vi "Notifier Test.vi"() -> ()   [LabVIEW 2021]
panel:
  in  "Any":bool
  out "size(s)":i32
  in  "name":string
  out "error out 3":errorcluster
  out "error out 2":errorcluster
  out "error out":errorcluster
  out "Iterations":i32
  in  "Add":bool
  in  "stop 2":bool
  in  "Send one":bool
  in  "Send two":bool
  in  "stop":bool
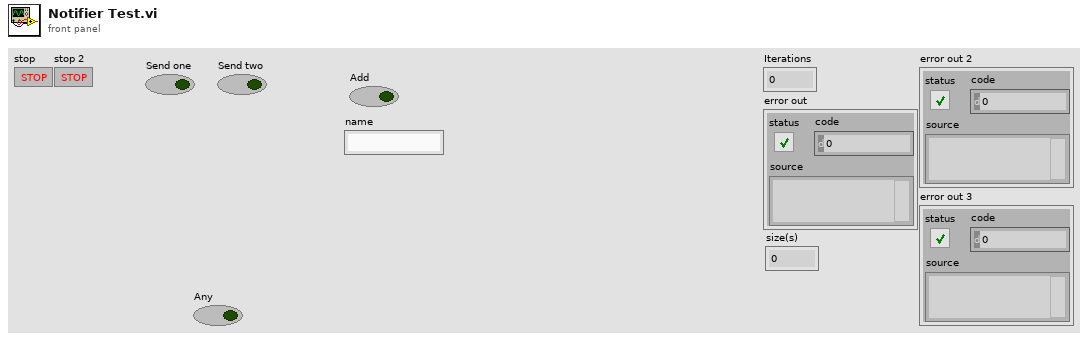
[diagram p1: front panel]
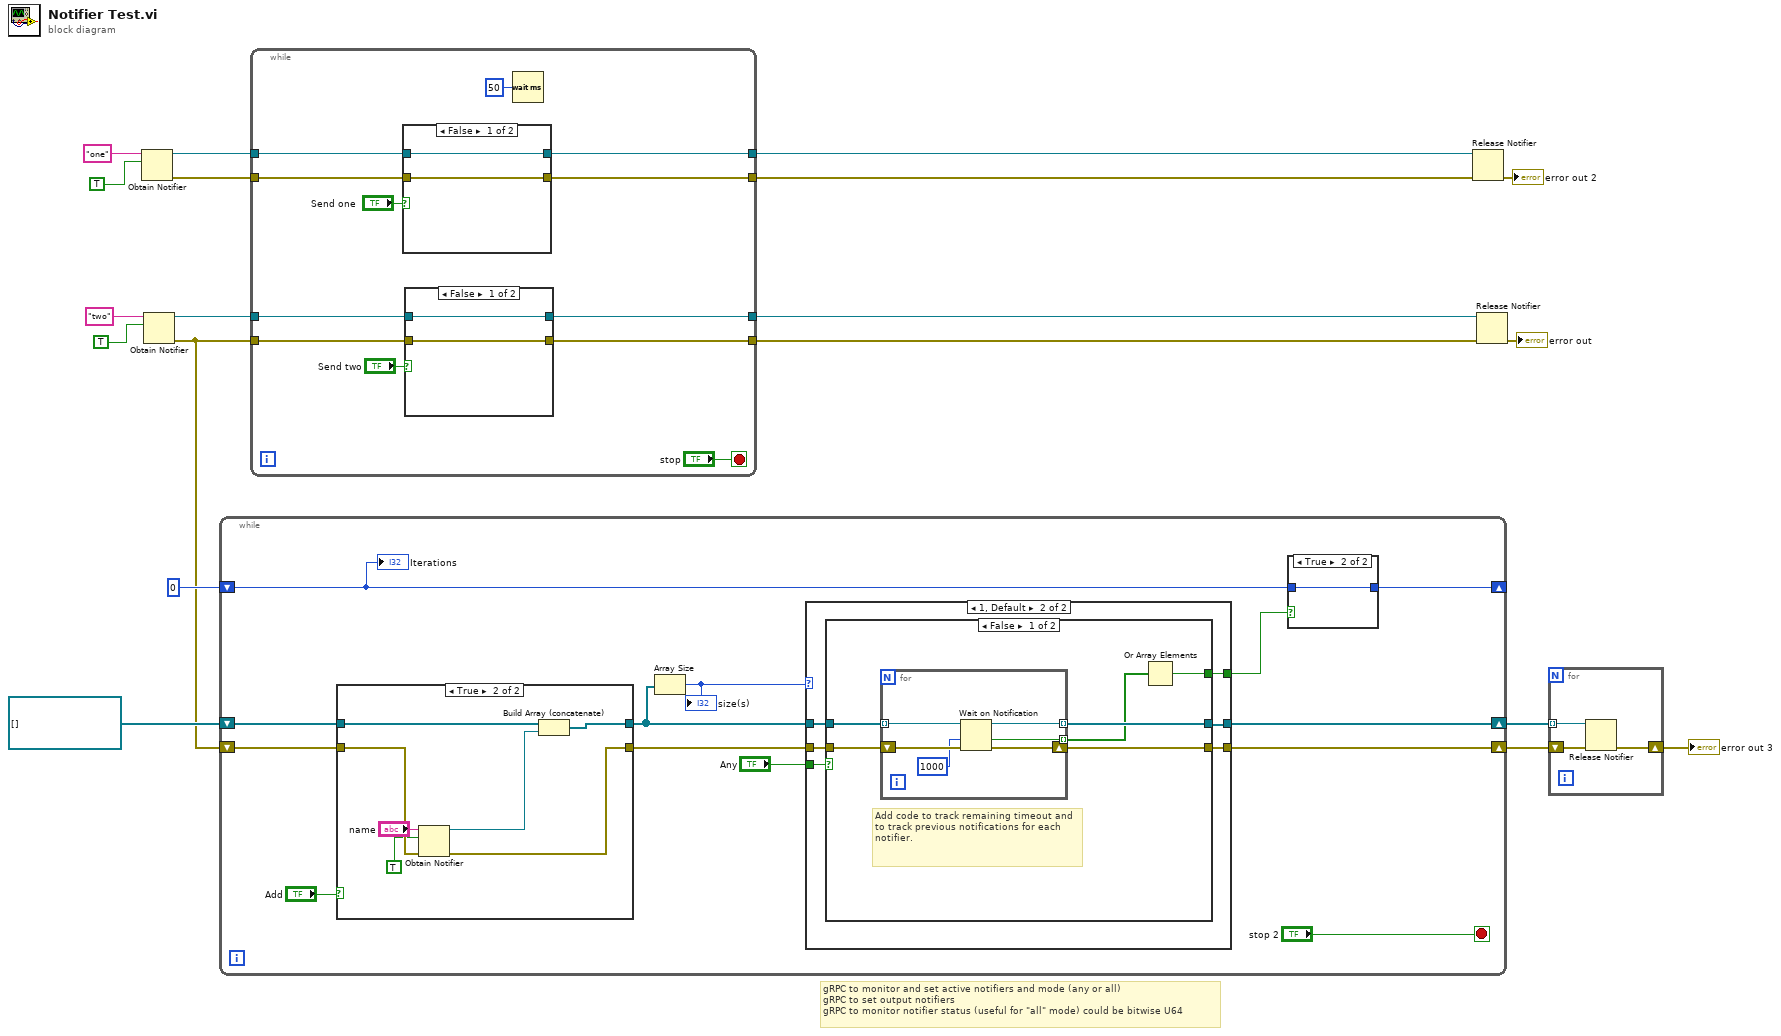
[diagram p0: block diagram]
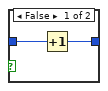
[diagram p2: hidden frame]
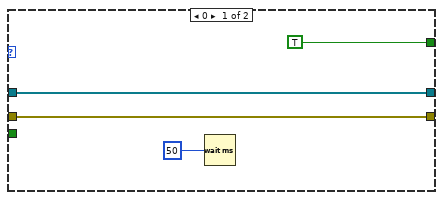
[diagram p3: hidden frame]
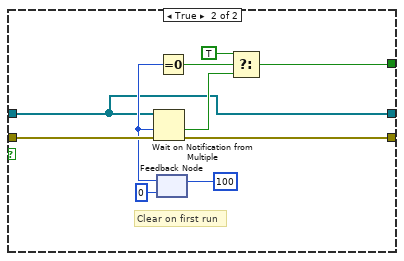
[diagram p4: hidden frame]
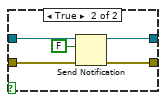
[diagram p6: hidden frame]
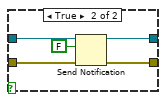
[diagram p7: hidden frame]
diagram:
  # "gRPC to monitor and set active notifiers and mode (any or all)\ngRPC to set output notifiers\ngRPC to monitor notifier status (useful for \"all\" mode) could be bitwise U64"
  n1 = Obtain Notifier(name (unnamed)="one", notification data type=TRUE) -> (notifier out=w14:refnum<notifier>, error out=w13:errorcluster)  [unwired: 2 in, 1 out]
  n2 = Obtain Notifier(name (unnamed)="two", notification data type=TRUE) -> (notifier out=w15:refnum<notifier>, error out=w3:errorcluster)  [unwired: 2 in, 1 out]
  n3 = while {
    shift-right: [w29] -> w6
    shift-left: refnum<notifier>[] [] ("notifiers") -> [w24]
    shift-right: [w21] -> _
    shift-left: 0 -> [w28]
    shift-right: [w27] -> w2
    shift-left: w3 -> [w25]
    stop <- "stop 2" stop-if-true
    n4 = case shown="True" "Add" {
      tunnel: w24 -> [w68 w74]
      tunnel: [w68 w73] -> w23
      tunnel: [w69 w71] -> w26
      tunnel: w25 -> [w69 w76]
      frame False {
      }
      frame True {
        n5 = Obtain Notifier(name (unnamed)="name", notification data type=TRUE, error in (no error)=w76) -> (notifier out=w70:refnum<notifier>, error out=w71:errorcluster)  [unwired: 1 in, 1 out]
        n6 = Build Array (concatenate)(w74, w70) -> (w73:refnum<notifier>[])
      }
    }
    n7 = Array Size(array=w23) -> (size(s)=w30:i32)
    "size(s)" <- w30
    n8 = case shown="1, Default" w30 {
      tunnel: w23 -> [w37 w43]
      tunnel: [w37 w40] -> w29
      tunnel: [w38 w45] -> w27
      tunnel: w26 -> [w38 w44]
      tunnel: [TRUE ("timed out?") w42] -> w22
      tunnel: "Any" -> [_ w41]
      frame 0 {
        n9 = Wait (ms)(milliseconds to wait=u32 50) -> ()  [unwired: 1 out]
      }
      frame 1, Default {
        n10 = case shown="False" w41 {
          tunnel: [w48 w67] -> w45
          tunnel: w44 -> [w50 w66]
          tunnel: w43 -> [w51 w58]
          tunnel: [w47 w59] -> w42
          tunnel: [w49 w58] -> w40
          frame False {
            # "Add code to track remaining timeout and to track previous notifications for each notifier."
            n11 = for {
              tunnel: w51 -> [w56] mode=indexing
              tunnel: [w57] -> w46 mode=indexing
              tunnel: [w55] -> w49 mode=indexing
              shift-right: [w53] -> w48
              shift-left: w50 -> [w54]
              n12 = Wait on Notification(notifier=w56, timeout in ms (-1)=1000, error in (no error)=w54) -> (notifier out=w55:refnum<notifier>, timed out?=w57:bool, error out=w53:errorcluster)  [unwired: 1 in, 1 out]
            }
            n13 = Or Array Elements(Boolean array=w46) -> (logical OR=w47:bool)
          }
          frame True {
            # "Clear on first run"
            n14 = feedback #1(0 ("timeout in ms (-1)")) -> (w63:i32)
            n15 = Wait on Notification from Multiple(0:w58, 2:w63, 3:w66) -> (10:w61:bool, 11:w67:errorcluster)  [unwired: 1 in, 2 out]
            n16 = feedback-in #1(100 ("timeout in ms (-1)")) -> ()
            n17 = Equal To 0?(x=w63) -> (x = 0?=w62:bool)
            n18 = Select(t=TRUE, s=w62, f=w61) -> (s? t:f=w59:bool)
          }
        }
      }
    }
    n19 = case shown="True" w22 {
      tunnel: w28 -> [w34 w35]
      tunnel: [w33 w35] -> w21
      frame False {
        n20 = Increment(x=w34) -> (x+1=w33:i32)
      }
      frame True {
      }
    }
    "Iterations" <- w28
  }
  n21 = while {
    tunnel: [w88] -> w12
    tunnel: [w87] -> w11
    tunnel: w15 -> [w84]
    tunnel: w3 -> [w83]
    tunnel: w14 -> [w80]
    tunnel: w13 -> [w81]
    tunnel: [w79] -> w10
    tunnel: [w78] -> w9
    stop <- "stop" stop-if-true
    n22 = case shown="False" "Send one" {
      tunnel: w80 -> [w90 w95]
      tunnel: w81 -> [w89 w94]
      tunnel: [w90 w93] -> w79
      tunnel: [w89 w92] -> w78
      frame False {
      }
      frame True {
        n23 = Send Notification(notification=FALSE, notifier=w95, error in (no error)=w94) -> (notifier out=w93:refnum<notifier>, error out=w92:errorcluster)
      }
    }
    n24 = case shown="False" "Send two" {
      tunnel: w84 -> [w97 w102]
      tunnel: w83 -> [w96 w101]
      tunnel: [w97 w100] -> w88
      tunnel: [w96 w99] -> w87
      frame False {
      }
      frame True {
        n25 = Send Notification(notification=FALSE, notifier=w102, error in (no error)=w101) -> (notifier out=w100:refnum<notifier>, error out=w99:errorcluster)
      }
    }
    n26 = Wait (ms)(milliseconds to wait=u32 50) -> ()  [unwired: 1 out]
  }
  n27 = Release Notifier(notifier=w10, error in (no error)=w9) -> (error out=→"error out 2":errorcluster)  [unwired: 1 in, 2 out]
  n28 = Release Notifier(notifier=w12, error in (no error)=w11) -> (error out=→"error out":errorcluster)  [unwired: 1 in, 2 out]
  n29 = for {
    tunnel: w6 -> [w105] mode=indexing
    shift-right: [w103] -> w1
    shift-left: w2 -> [w104]
    n30 = Release Notifier(notifier=w105, error in (no error)=w104) -> (error out=w103:errorcluster)  [unwired: 1 in, 2 out]
  }
  "error out 3" <- w1
